vi "8.2.SSD1306_64x48_Example_Frame.vi"   [LabVIEW 2014]
uses:
  QwaveSys_Interface/QwaveSys_Interface.lvlib
  <vilib>/Aledyne-TSXperts/Arduino Compatible Compiler for LabVIEW/Arduino Compatible Compiler for LabVIEW.lvlib
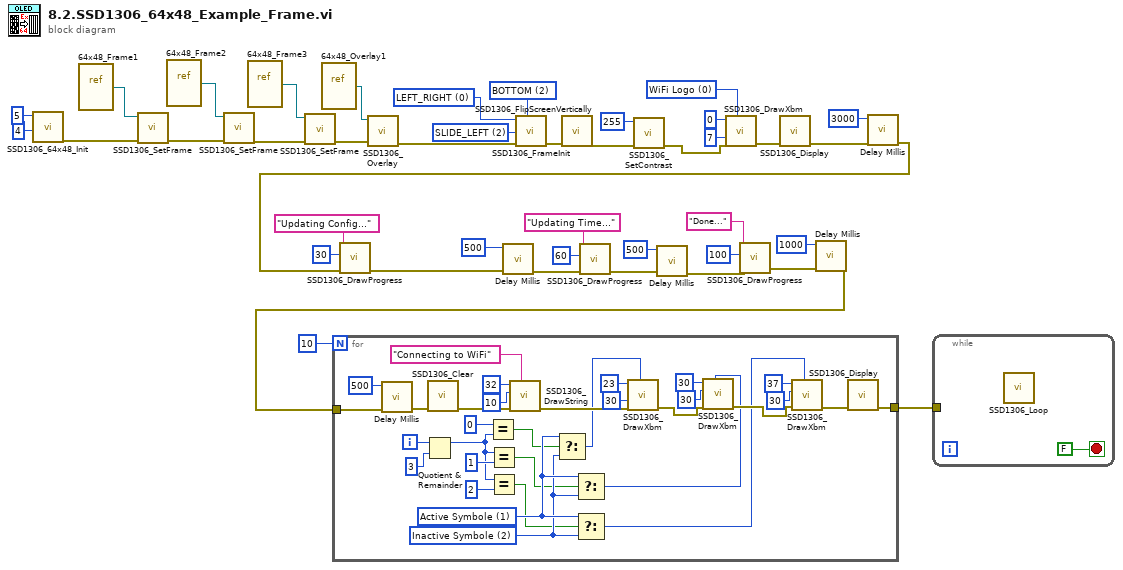
[diagram p0: block diagram]
diagram:
  w4 = u8 2 items=["SLIDE_UP", "SLIDE_DOWN", "SLIDE_LEFT", "SLIDE_RIGHT"] ("Frame Animation")
  w5 = u8 0 items=["LEFT_RIGHT", "RIGHT_LEFT"] ("Indicator Direction")
  w6 = u8 2 items=["TOP", "RIGHT", "BOTTOM", "LEFT"] ("Indicator Position")
  w37 = u16 0 items=["WiFi Logo", "Active Symbole", "Inactive Symbole"] ("xbm")
  n1 = call "SSD1306_64x48_Init.vi"("SDA"=u8 4, "SCL"=u8 5) -> ("error out"=w14:errorcluster)  [unwired: 9 in]
  n2 = vi-ref "64x48_Frame1.vi"() -> (w42:refnum<vi>)
  n3 = call "SSD1306_SetFrame.vi"("error in (no error)"=w14, "VI Frame"=w42) -> ("error out"=w40:errorcluster)  [unwired: 9 in]
  n4 = vi-ref "64x48_Frame2.vi"() -> (w41:refnum<vi>)
  n5 = call "SSD1306_SetFrame.vi"("error in (no error)"=w40, "VI Frame"=w41) -> ("error out"=w12:errorcluster)  [unwired: 9 in]
  n6 = vi-ref "64x48_Frame3.vi"() -> (w13:refnum<vi>)
  n7 = call "SSD1306_SetFrame.vi"("error in (no error)"=w12, "VI Frame"=w13) -> ("error out"=w11:errorcluster)  [unwired: 9 in]
  n8 = vi-ref "64x48_Overlay1.vi"() -> (w9:refnum<vi>)
  n9 = call "SSD1306_Overlay.vi"("error in (no error)"=w11, "VI Overlay"=w9) -> ("error out"=w8:errorcluster)  [unwired: 9 in]
  n10 = call "SSD1306_FrameInit.vi"("Indicator Position"=w6, "error in (no error)"=w8, "Frame Animation"=w4, "Indicator Direction"=w5) -> ("error out"=w7:errorcluster)  [unwired: 7 in]
  n11 = call "SSD1306_FlipScreenVertically.vi"("error in (no error)"=w7) -> ("error out"=w10:errorcluster)  [unwired: 10 in]
  n12 = call "SSD1306_SetContrast.vi"("error in (no error)"=w10, "contrast"=u8 255) -> ("error out"=w32:errorcluster)  [unwired: 9 in]
  n13 = call "SSD1306_DrawXbm.vi"("xbm"=w37, "error in (no error)"=w32, "y"=u8 7, "x"=u8 0) -> ("error out"=w34:errorcluster)  [unwired: 7 in]
  n14 = call "SSD1306_Display.vi"("error in (no error)"=w34) -> ("error out"=w31:errorcluster)  [unwired: 10 in]
  n15 = call <vilib>:"Delay Millis.vi"("error in (no error)"=w31, "delay"=u32 3000) -> ("error out"=w18:errorcluster)  [unwired: 9 in]
  n16 = call "SSD1306_DrawProgress.vi"("error in (no error)"=w18, "percentage"=u8 30 ("%"), "String"="Updating Config...") -> ("error out"=w21:errorcluster)  [unwired: 8 in]
  n17 = call <vilib>:"Delay Millis.vi"("error in (no error)"=w21, "delay"=u32 500) -> ("error out"=w19:errorcluster)  [unwired: 9 in]
  n18 = call "SSD1306_DrawProgress.vi"("error in (no error)"=w19, "percentage"=u8 60 ("%"), "String"="Updating Time...") -> ("error out"=w29:errorcluster)  [unwired: 8 in]
  n19 = call <vilib>:"Delay Millis.vi"("error in (no error)"=w29, "delay"=u32 500) -> ("error out"=w28:errorcluster)  [unwired: 9 in]
  n20 = call "SSD1306_DrawProgress.vi"("error in (no error)"=w28, "percentage"=u8 100 ("%"), "String"="Done...") -> ("error out"=w15:errorcluster)  [unwired: 8 in]
  n21 = call <vilib>:"Delay Millis.vi"("error in (no error)"=w15, "delay"=u32 1000) -> ("error out"=w16:errorcluster)  [unwired: 9 in]
  n22 = for {
    N: 10 -> [_]
    tunnel: [w46] -> w3
    tunnel: w16 -> [w45]
    i -> [w74]
    w54 = u16 2 items=["WiFi Logo", "Active Symbole", "Inactive Symbole"] ("xbm")
    w55 = u16 1 items=["WiFi Logo", "Active Symbole", "Inactive Symbole"] ("xbm")
    n23 = call <vilib>:"Delay Millis.vi"("error in (no error)"=w45, "delay"=u32 500) -> ("error out"=w72:errorcluster)  [unwired: 9 in]
    n24 = Quotient & Remainder(x=w74, y=3) -> (x-y*floor(x/y)=w44:i32)  [unwired: 1 out]
    n25 = call "SSD1306_Clear.vi"("error in (no error)"=w72) -> ("error out"=w69:errorcluster)  [unwired: 10 in]
    n26 = Equal?(x=0, y=w44) -> (x = y?=w53:bool)
    n27 = Equal?(x=w44, y=1) -> (x = y?=w52:bool)
    n28 = Equal?(x=w44, y=2) -> (x = y?=w51:bool)
    n29 = call "SSD1306_DrawString.vi"("String"="Connecting to WiFi", "error in (no error)"=w69, "y"=u8 10, "x"=u8 32) -> ("error out"=w68:errorcluster)  [unwired: 7 in]
    n30 = Select(t=w55, s=w53, f=w54) -> (s? t:f=w49:u16)
    n31 = Select(t=w55, s=w52, f=w54) -> (s? t:f=w50:u16)
    n32 = Select(t=w55, s=w51, f=w54) -> (s? t:f=w48:u16)
    n33 = call "SSD1306_DrawXbm.vi"("xbm"=w49, "error in (no error)"=w68, "y"=u8 30, "x"=u8 23) -> ("error out"=w60:errorcluster)  [unwired: 7 in]
    n34 = call "SSD1306_DrawXbm.vi"("xbm"=w50, "error in (no error)"=w60, "y"=u8 30, "x"=u8 30) -> ("error out"=w59:errorcluster)  [unwired: 7 in]
    n35 = call "SSD1306_DrawXbm.vi"("xbm"=w48, "error in (no error)"=w59, "y"=u8 30, "x"=u8 37) -> ("error out"=w47:errorcluster)  [unwired: 7 in]
    n36 = call "SSD1306_Display.vi"("error in (no error)"=w47) -> ("error out"=w46:errorcluster)  [unwired: 10 in]
  }
  n37 = while {
    tunnel: w3 -> [_]
    stop <- FALSE stop-if-true
    n38 = call "SSD1306_Loop.vi"() -> ()  [unwired: 11 in, 1 out]
  }
